vi "Fire-Sequence.vi"(2 "La Fire at will?":bool) -> ()   [LabVIEW 2012]
uses:
  BotStatus.vi
  Motors Values.vi
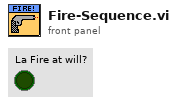
[diagram p1: front panel]
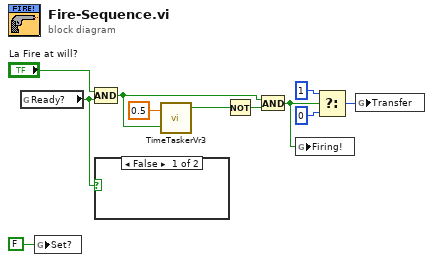
[diagram p0: block diagram]
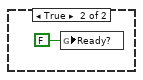
[diagram p2: hidden frame]
diagram:
  n1 = global read "BotStatus.vi" "Ready?"() -> (w1:bool)
  n2 = global write "BotStatus.vi" "Set?"(FALSE ("Set?")) -> ()
  n3 = Compound Arithmetic op=AND("La Fire at will?", w1) -> (w4:bool)
  n4 = case shown="False" w1 {
    frame False {
    }
    frame True {
      n5 = global write "BotStatus.vi" "Ready?"(FALSE ("Set?")) -> ()
    }
  }
  n6 = call "TimeTaskerVr3.vi"("Delay(sec)"=0.5, "Start Counting?"=w4) -> ("TimePast?"=w10:bool)  [unwired: 2 out]
  n7 = Not(x=w10) -> (.not. x?=w9:bool)
  n8 = And(x=w4, y=w9) -> (x .and. y?=w5:bool)
  n9 = global write "BotStatus.vi" "Firing!"(w5) -> ()
  n10 = Select(t=1, s=w5, f=0) -> (s? t:f=w7:i32)
  n11 = global write "Motors Values.vi" "Transfer"(w7) -> ()
